vi "piezoReadClose.vi"   [LabVIEW 2017]
uses:
  globalDevices.vi
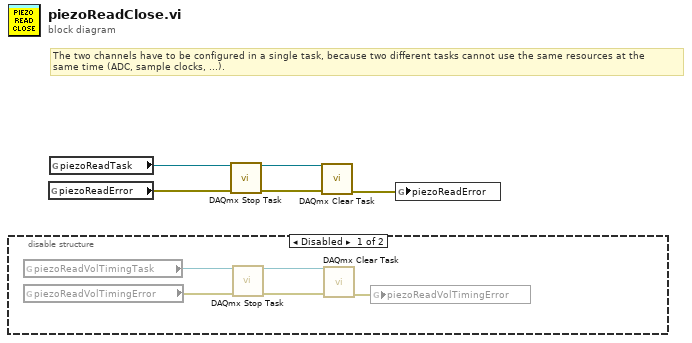
[diagram p0: block diagram]
diagram:
  # "The two channels have to be configured in a single task, because two different tasks cannot use the same resources at the\nsame time (ADC, sample clocks, ...)."
  n1 = disable-structure shown="Disabled" {
    frame Disabled {
      n2 = global read "globalDevices.vi" "piezoReadVolTimingTask"() -> (w8:refnum<k21>)
      n3 = global read "globalDevices.vi" "piezoReadVolTimingError"() -> (w9:errorcluster)
      n4 = call <vilib>:"DAQmx Stop Task.vi"("task/channels in"=w8, "error in"=w9) -> ("task out"=w6:refnum<k21>, "error out"=w7:errorcluster)  [unwired: 12 in]
      n5 = call <vilib>:"DAQmx Clear Task.vi"("task in"=w6, "error in"=w7) -> ("error out"=w10:errorcluster)  [unwired: 13 in]
      n6 = global write "globalDevices.vi" "piezoReadVolTimingError"(w10) -> ()
    }
    frame Enabled {
    }
  }
  n7 = global read "globalDevices.vi" "piezoReadError"() -> (w2:errorcluster)
  n8 = global read "globalDevices.vi" "piezoReadTask"() -> (w3:refnum<k21>)
  n9 = call <vilib>:"DAQmx Stop Task.vi"("task/channels in"=w3, "error in"=w2) -> ("task out"=w5:refnum<k21>, "error out"=w4:errorcluster)  [unwired: 12 in]
  n10 = call <vilib>:"DAQmx Clear Task.vi"("task in"=w5, "error in"=w4) -> ("error out"=w1:errorcluster)  [unwired: 13 in]
  n11 = global write "globalDevices.vi" "piezoReadError"(w1) -> ()
